vi "GetSetMotorAxisValue.vi"(8 "set? (T)":bool=TRUE, 9 "pos":dbl, 10 "axis":T1, 11 "Motorpos in":T2) -> (2 "pos (out)":dbl, 3 "Motorpos out":T2)   [LabVIEW 2011]
uses:
  MotorPosType.ctl
  Typedefs/XYf.ctl
  MotorAxisEnum.ctl
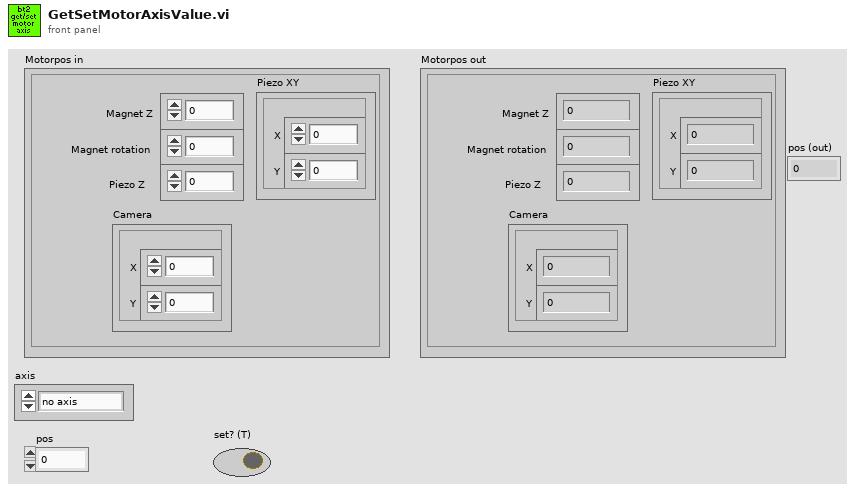
[diagram p1: front panel]
types:
  T1 = typedef "MotorAxisEnum.ctl" = enum16{"no axis", "magrot", "magpos", "px", "py", "pz", "camx", "camy"}
  T2 = typedef "MotorPosType.ctl" = cluster{"Magnet Z":dbl, "Magnet rotation":dbl, "Camera":T3, "Piezo XY":T3, "Piezo Z":dbl}
  T3 = typedef "XYf.ctl" = cluster{"X":sgl, "Y":sgl}
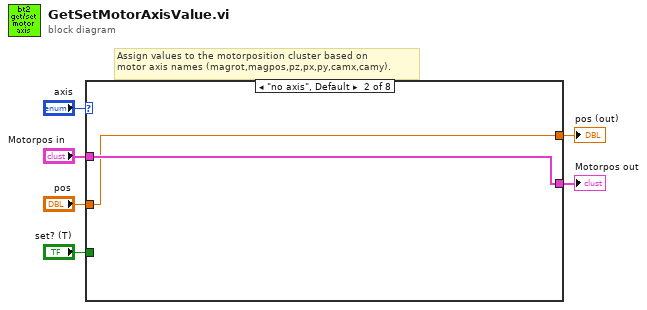
[diagram p0: block diagram]
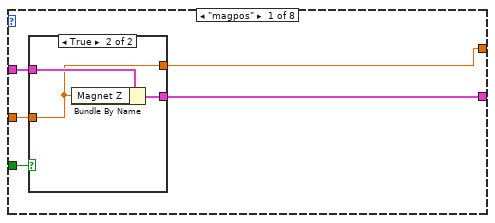
[diagram p2: hidden frame]
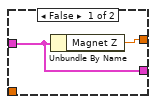
[diagram p3: hidden frame]
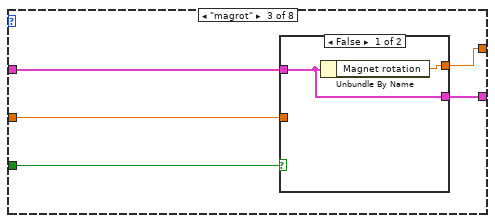
[diagram p4: hidden frame]
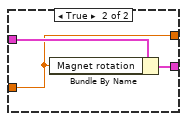
[diagram p5: hidden frame]
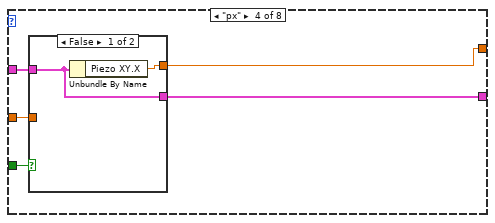
[diagram p6: hidden frame]
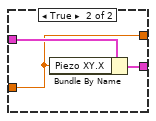
[diagram p7: hidden frame]
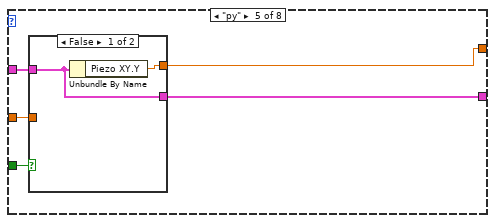
[diagram p8: hidden frame]
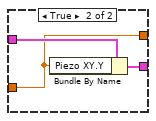
[diagram p9: hidden frame]
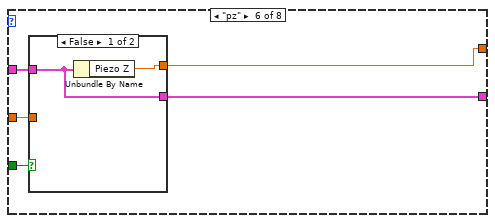
[diagram p10: hidden frame]
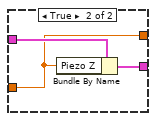
[diagram p11: hidden frame]
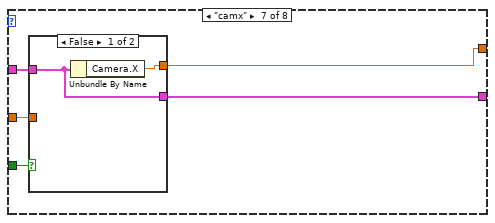
[diagram p12: hidden frame]
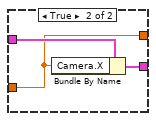
[diagram p13: hidden frame]
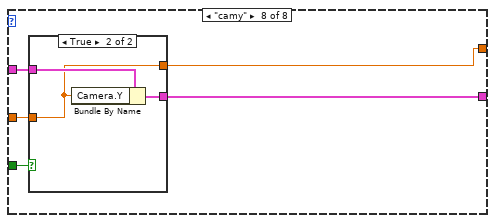
[diagram p14: hidden frame]
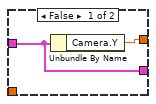
[diagram p15: hidden frame]
diagram:
  # "Assign values to the motorposition cluster based on\nmotor axis names (magrot,magpos,pz,px,py,camx,camy)."
  n1 = case shown="\"no axis\", Default" "axis" {
    tunnel: "Motorpos in" -> [w11 w18 w23 w33 w43 w52 w63 w73]
    tunnel: [w10 w18 w22 w32 w42 w53 w62 w72] -> w5
    tunnel: "pos" -> [w9 w17 w21 w31 w41 w51 w61 w71]
    tunnel: "set? (T)" -> [w8 _ w20 w29 w40 w50 w60 w70]
    tunnel: [w7 w17 w19 w30 w39 w49 w59 w69] -> w1
    frame "magpos" {
      n2 = case shown="True" w8 {
        tunnel: w11 -> [w12 w16]
        tunnel: [w12 w15] -> w10
        tunnel: w9 -> [_ w14]
        tunnel: [w13 w14] -> w7
        frame False {
          n3 = Unbundle By Name(w12) -> ("Magnet Z"=w13:dbl)
        }
        frame True {
          n4 = Bundle By Name(cluster=w16, "Magnet Z"=w14) -> (w15:T2)
        }
      }
    }
    frame "no axis", Default {
    }
    frame "magrot" {
      n5 = case shown="False" w20 {
        tunnel: w23 -> [w24 w28]
        tunnel: [w24 w27] -> w22
        tunnel: w21 -> [_ w26]
        tunnel: [w25 w26] -> w19
        frame False {
          n6 = Unbundle By Name(w24) -> ("Magnet rotation"=w25:dbl)
        }
        frame True {
          n7 = Bundle By Name(cluster=w28, "Magnet rotation"=w26) -> (w27:T2)
        }
      }
    }
    frame "px" {
      n8 = case shown="False" w29 {
        tunnel: w33 -> [w34 w38]
        tunnel: [w34 w37] -> w32
        tunnel: w31 -> [_ w36]
        tunnel: [w35 w36] -> w30
        frame False {
          n9 = Unbundle By Name(w34) -> ("Piezo XY.X"=w35:sgl)
        }
        frame True {
          n10 = Bundle By Name(cluster=w38, "Piezo XY.X"=w36) -> (w37:T2)
        }
      }
    }
    frame "py" {
      n11 = case shown="False" w40 {
        tunnel: w43 -> [w44 w48]
        tunnel: [w44 w47] -> w42
        tunnel: w41 -> [_ w46]
        tunnel: [w45 w46] -> w39
        frame False {
          n12 = Unbundle By Name(w44) -> ("Piezo XY.Y"=w45:sgl)
        }
        frame True {
          n13 = Bundle By Name(cluster=w48, "Piezo XY.Y"=w46) -> (w47:T2)
        }
      }
    }
    frame "pz" {
      n14 = case shown="False" w50 {
        tunnel: [w54 w58] -> w53
        tunnel: w52 -> [w54 w57]
        tunnel: w51 -> [_ w56]
        tunnel: [w55 w56] -> w49
        frame False {
          n15 = Unbundle By Name(w54) -> ("Piezo Z"=w55:dbl)
        }
        frame True {
          n16 = Bundle By Name(cluster=w57, "Piezo Z"=w56) -> (w58:T2)
        }
      }
    }
    frame "camx" {
      n17 = case shown="False" w60 {
        tunnel: w63 -> [w64 w68]
        tunnel: [w64 w67] -> w62
        tunnel: w61 -> [_ w66]
        tunnel: [w65 w66] -> w59
        frame False {
          n18 = Unbundle By Name(w64) -> ("Camera.X"=w65:sgl)
        }
        frame True {
          n19 = Bundle By Name(cluster=w68, "Camera.X"=w66) -> (w67:T2)
        }
      }
    }
    frame "camy" {
      n20 = case shown="True" w70 {
        tunnel: w73 -> [w74 w78]
        tunnel: [w74 w77] -> w72
        tunnel: w71 -> [_ w76]
        tunnel: [w75 w76] -> w69
        frame False {
          n21 = Unbundle By Name(w74) -> ("Camera.Y"=w75:sgl)
        }
        frame True {
          n22 = Bundle By Name(cluster=w78, "Camera.Y"=w76) -> (w77:T2)
        }
      }
    }
  }
  "Motorpos out" <- w5
  "pos (out)" <- w1
